vi "Collatz Sequence Length.vi"(11 "n":u64) -> (3 "Sequence Length":i32)   [LabVIEW 2013, in "Problem 14.lvlib"]
uses:
  Problem 14.lvlib
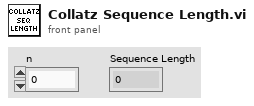
[diagram p1: front panel]
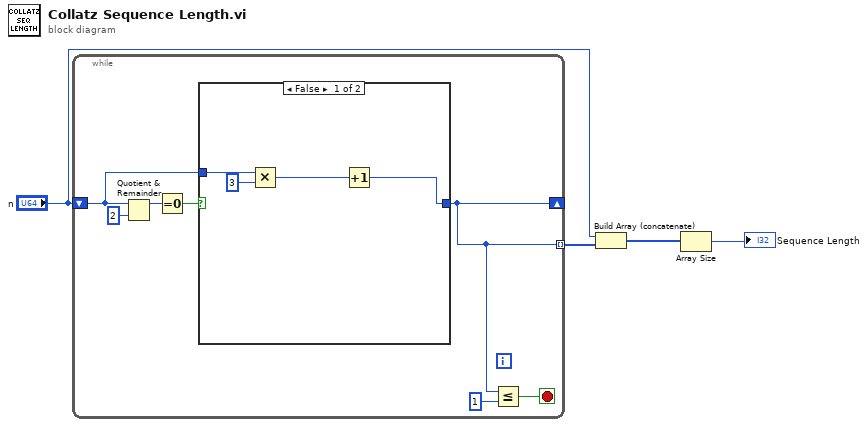
[diagram p0: block diagram]
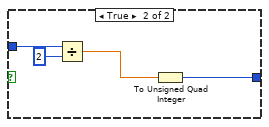
[diagram p2: hidden frame]
diagram:
  n1 = while {
    shift-right: [w5] -> _
    shift-left: "n" -> [w6]
    tunnel: [w5] -> w4 mode=indexing
    stop <- w8 stop-if-true
    n2 = Quotient & Remainder(x=w6, y=u64 2) -> (x-y*floor(x/y)=w10:u64)  [unwired: 1 out]
    n3 = Equal To 0?(x=w10) -> (x = 0?=w9:bool)
    n4 = case shown="False" w9 {
      tunnel: w6 -> [w15 w19]
      tunnel: [w12 w16] -> w5
      frame False {
        n5 = Multiply(x=w15, y=u64 3) -> (x*y=w13:u64)
        n6 = Increment(x=w13) -> (x+1=w12:u64)
      }
      frame True {
        n7 = Divide(x=w19, y=u64 2) -> (x/y=w17:dbl)
        n8 = To Unsigned Quad Integer(1:w17) -> (0:w16:u64)
      }
    }
    n9 = Less Or Equal?(x=w5, y=u64 1) -> (x <= y?=w8:bool)
  }
  n10 = Build Array (concatenate)("n", w4) -> (w2:u64[])
  n11 = Array Size(array=w2) -> (size(s)=→"Sequence Length":i32)
